vi "DrawBeam.vi"(3 "Color":u32(colorbox)=16716800, 4 "Beam radius":sgl=0.02, 5 "Point":dbl[](array[numeric])=[0.0, 0.0, 0.0], 6 "Name":string="Axis X") -> (1 "Beam":refnum<vi>)   [LabVIEW 2024]
uses:
  <vilib>/picture/3D Picture Control/Object/Create Object (drawable).vi
  <vilib>/picture/3D Picture Control/NI_3D Picture Control.lvlib
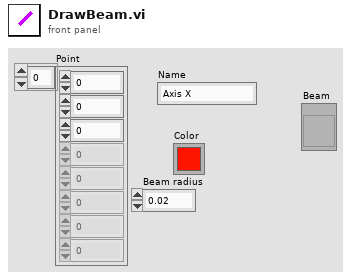
[diagram p1: front panel]
types:
  T1 = cluster{"Red":sgl, "Green":sgl, "Blue":sgl, "Alpha":sgl}
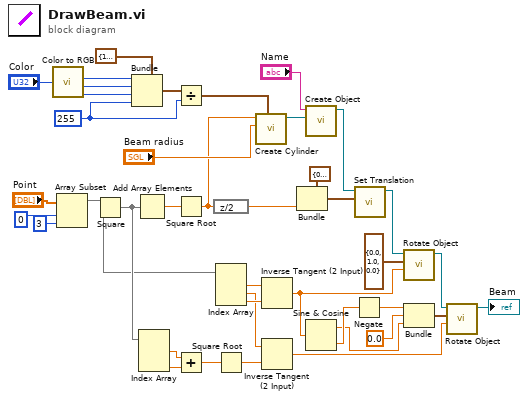
[diagram p0: block diagram]
diagram:
  w6 = 255
  n1 = call <vilib>:"Color to RGB.vi"("Color"="Color") -> ("R"=w10:u8, "G"=w9:u8, "B"=w8:u8)  [unwired: 1 out]
  n2 = Array Subset(array="Point", index=0, length=3) -> (w3:dbl[])
  n3 = Square(x=w3) -> (x^2=w19:dbl[])
  n4 = Bundle(cluster=T1 {"Red"=1.0, "Green"=0.0, "Blue"=0.0, "Alpha"=1.0} ("Color"), "Red"=w10, "Green"=w9, "Blue"=w8, "Alpha"=w6) -> (w7:T1)
  n5 = Add Array Elements(numeric array=w19) -> (sum=w38:dbl)
  n6 = Index Array(array=w19) -> (element #1=w18:dbl, element #3=w17:dbl)  [unwired: 3 in, 1 out]
  n7 = Divide(x=w7, y=w6) -> (x/y=w4:T1)
  n8 = Square Root(x=w38) -> (sqrt(x)=w31:dbl)
  n9 = Add(x=w18, y=w17) -> (x+y=w16:dbl)
  n10 = expression code="z/2"(w31) -> (w30:dbl)
  n11 = Index Array(array=w3) -> (element #1=w21:dbl, element #2=w15:dbl, element #3=w20:dbl)  [unwired: 3 in]
  n12 = Square Root(x=w16) -> (sqrt(x)=w14:dbl)
  n13 = call <vilib>:"Create Cylinder.vi"("Color"=w4, "Radius"="Beam radius", "Height"=w31) -> ("New Cylinder Refnum"=w36:refnum<vi>)  [unwired: 7 in, 1 out]
  n14 = Inverse Tangent (2 Input)(1:w20, 2:w21) -> (0:w12:dbl)
  n15 = Inverse Tangent (2 Input)(1:w14, 2:w15) -> (0:w13:dbl)
  n16 = Bundle(cluster=cluster{"X":sgl, "Y":sgl, "Z":sgl} {"X"=0.0, "Y"=0.0, "Z"=1.0} ("Translation"), "Z"=w30) -> (w32:cluster{"X":sgl, "Y":sgl, "Z":sgl})  [unwired: 2 in]
  n17 = call-poly <vilib>:"Create Object.vi"("Geometry"=w36, "Name"="Name") -> ("Scene:New Object"=w34:refnum<vi>)  [unwired: 8 in, 1 out]
  n18 = Sine & Cosine(0:w12) -> (1:w25:dbl, 2:w27:dbl)
  n19 = Negate(x=w27) -> (-x=w26:dbl)
  n20 = call <vilib>:"Set Translation.vi"("Translation"=w32, "Scene Object"=w34) -> ("Translated Object"=w29:refnum<vi>)  [unwired: 8 in, 1 out]
  n21 = call <vilib>:"Rotate Object.vi"("Angle"=w12, "Axis"=cluster{"X":sgl, "Y":sgl, "Z":sgl} {"X"=0.0, "Y"=1.0, "Z"=0.0}, "Scene.Object In"=w29) -> ("Scene.Object Out"=w28:refnum<vi>)  [unwired: 7 in, 1 out]
  n22 = Bundle(w26, "Angle"=sgl 0.0, w25) -> (w23:cluster{dbl, "Angle":sgl, dbl})  [unwired: 1 in]
  n23 = call <vilib>:"Rotate Object.vi"("Angle"=w13, "Axis"=w23, "Scene.Object In"=w28) -> ("Scene.Object Out"=→"Beam":refnum<vi>)  [unwired: 7 in, 1 out]
